vi "Database_UUT - Add UUT.vi"() -> ()   [LabVIEW 2017]
uses:
  Database_UUT_class/TypeDefs/Datatype.ctl
  Database_UUT_class/Database_UUT.lvclass
panel:
  in  "View Part Number":bool
  in  "Part Number:":string="700-001-25"
  in  "Property Values":string[](array[string])
  in  "Datatype":T1[](array[typedef])=[enum."Double", enum."Int32", enum."Double", enum."Double", enum."Double", enum."Double"]
  in  "Property Labels":string[](array[string])=["Rated Current (A)", "Overload Current (%)", "Lower Trip Limit (s)", "Upper Trip Limit (s)", "Maximum Trip Limit (s)", "Cooling Time (s)"]
  in  "View Database":bool
  in  "Quit Program":bool
  in  "Remove From Database":bool
  in  "Verify Path":bool
  in  "Submit Into Database":bool
  in  "TDMS Database File Name:":string="Database"
  in  "Filepath to Directory of Database:":path=path "C:/Users/Test-Eng/Desktop/ATE Development Programing/Database"
  # "TDMS Database Tool Boss 4000"
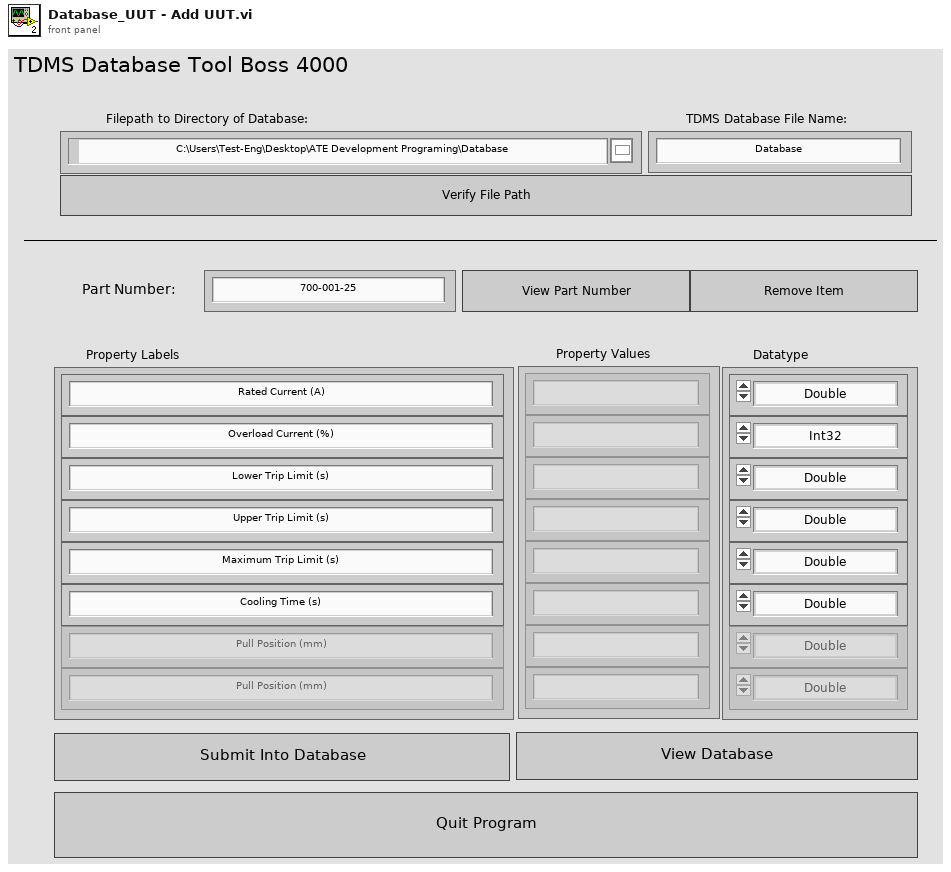
[diagram p1: front panel]
types:
  T1 = typedef "Database_UUT.lvclass/Datatype.ctl" = enum16{"Double", "Int32", "Text String", "Bool (0 or 1)"}
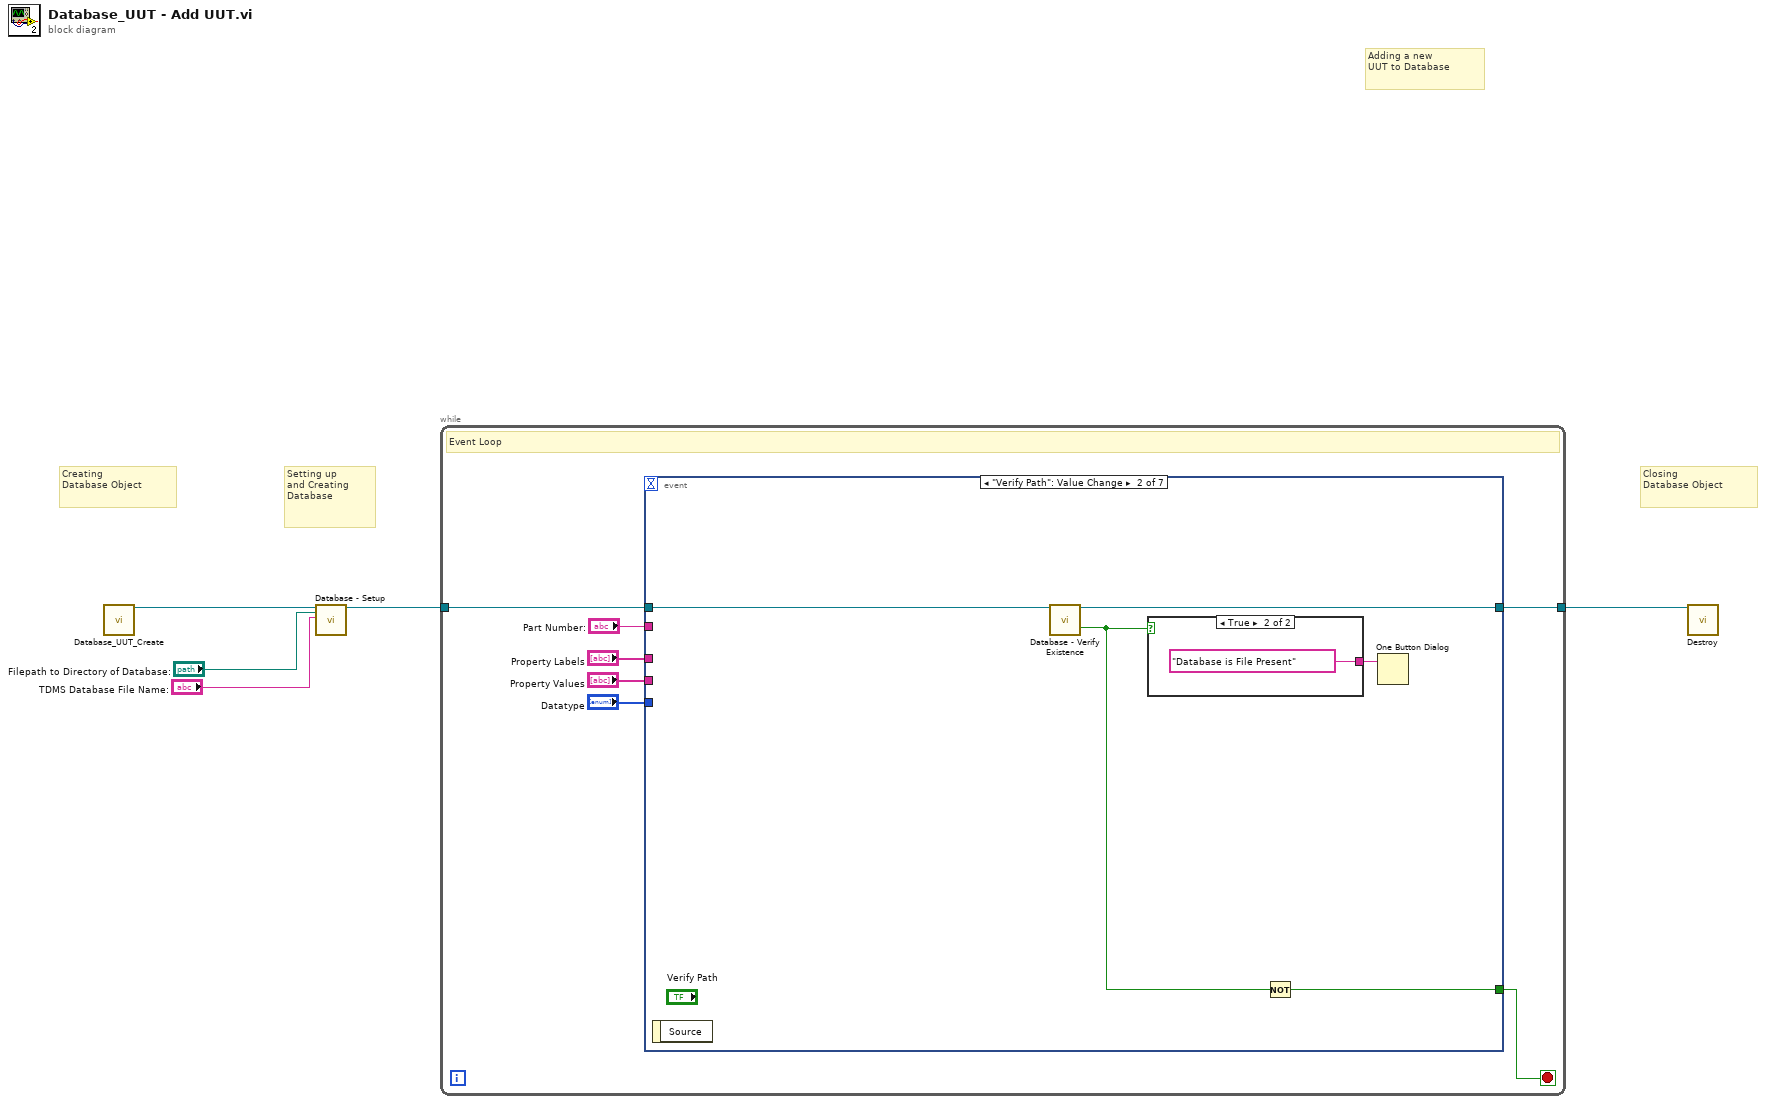
[diagram p0: block diagram]
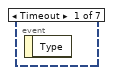
[diagram p2: hidden frame]
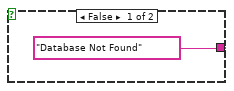
[diagram p3: hidden frame]
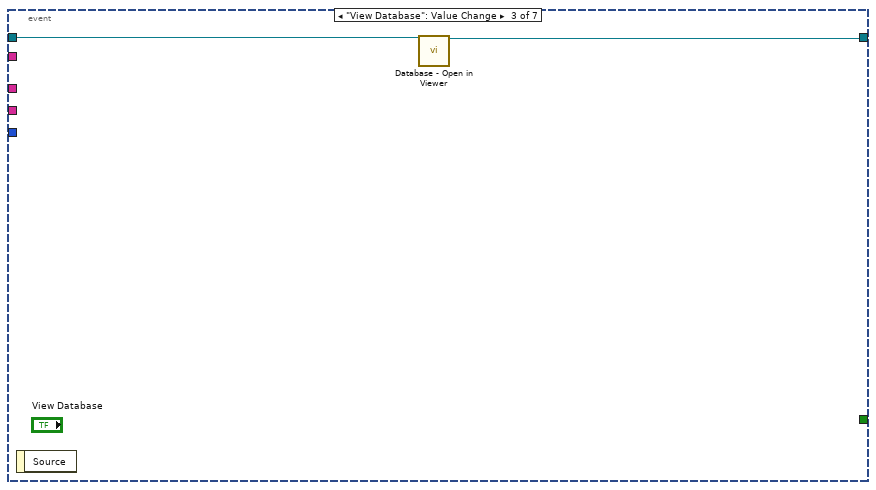
[diagram p4: hidden frame]
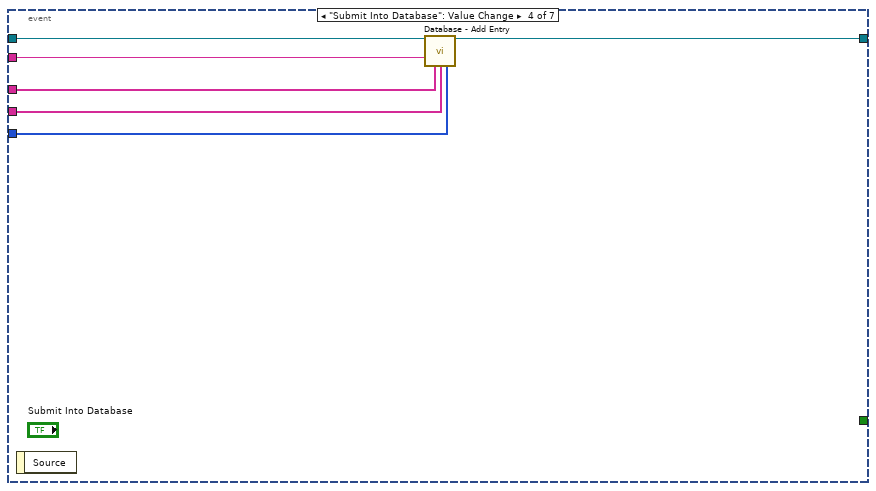
[diagram p5: hidden frame]
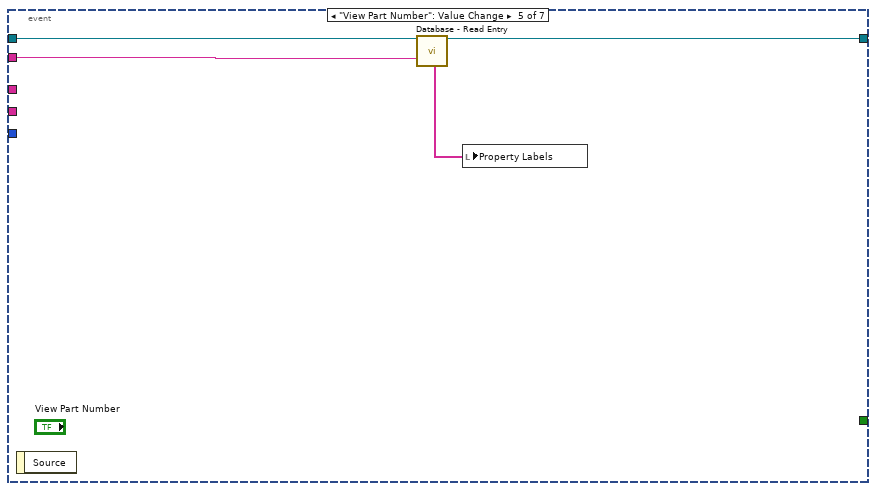
[diagram p6: hidden frame]
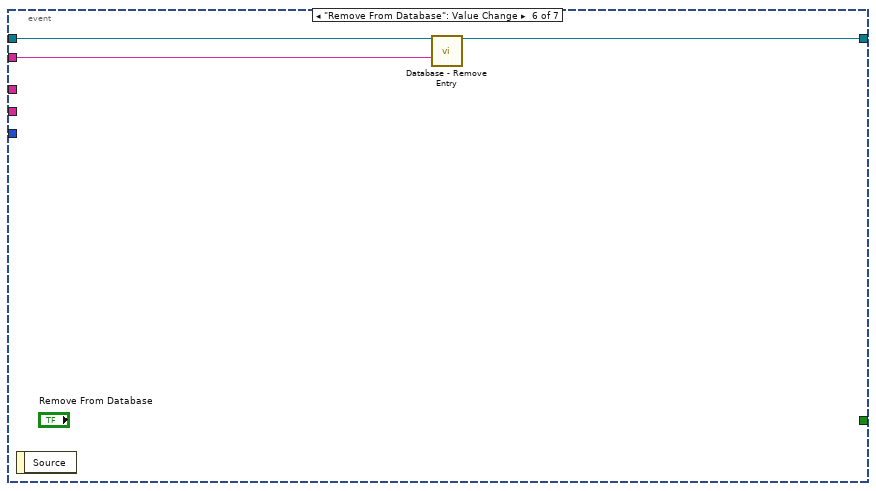
[diagram p7: hidden frame]
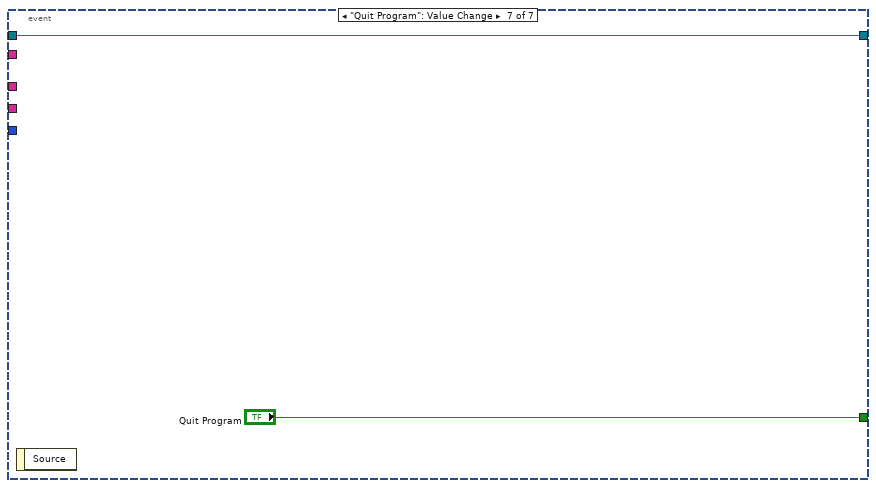
[diagram p8: hidden frame]
diagram:
  # "Closing\nDatabase Object"
  # "Adding a new\nUUT to Database"
  # "Setting up\nand Creating\nDatabase"
  # "Creating\nDatabase Object"
  n1 = call "Database_UUT_Create.vi"() -> ("reference out"=w5:refnum<class "Database_UUT.lvclass">)  [unwired: 18 in, 1 out]
  n2 = call-dynamic "Database - Setup.vi"("reference in"=w5, "Filepath to Directory of Database"="Filepath to Directory of Database:", "Database Name"="TDMS Database File Name:") -> ("reference out"=w2:refnum<class "Database_UUT.lvclass">)  [unwired: 14 in, 2 out]
  n3 = while {
    tunnel: w2 -> [w11]
    tunnel: [w12] -> w1
    stop <- w10 stop-if-true
    # "Event Loop"
    n4 = event shown="[1] \"Verify Path\": Value Change" {
      selector: _ -> [_ _ _ _ _ _ _]
      dyn-events: _ -> [_ _ _ _ _ _ _]
      timeout: _ -> [_ _ _ _ _ _ _]
      tunnel: [_ w16 w20 w26 w30 w34 w35] -> w12
      tunnel: w11 -> [_ w17 w21 w27 w31 w33 w35]
      tunnel: [_ w13 _ _ _ _ "Quit Program"] -> w10
      tunnel: "Part Number:" -> [_ _ _ w25 w29 w32 _]
      tunnel: "Datatype" -> [_ _ _ w24 _ _ _]
      tunnel: "Property Values" -> [_ _ _ w23 _ _ _]
      tunnel: "Property Labels" -> [_ _ _ w22 _ _ _]
      event Timeout {
        n5 = event-data() -> ()  [unwired: 1 in, 1 out]
      }
      event "Verify Path": Value Change {
        n6 = event-data() -> ()  [unwired: 1 in, 1 out]
        n7 = call-dynamic "Database - Verify Existence.vi"("reference in"=w17) -> ("reference out"=w16:refnum<class "Database_UUT.lvclass">, "File Exists/Verified"=w14:bool)  [unwired: 16 in, 1 out]
        n8 = case shown="True" w14 {
          tunnel: ["Database Not Found" "Database is File Present"] -> w15
          frame False {
          }
          frame True {
          }
        }
        n9 = Not(x=w14) -> (.not. x?=w13:bool)
        n10 = One Button Dialog(message=w15) -> ()  [unwired: 1 in, 1 out]
      }
      event "View Database": Value Change {
        n11 = event-data() -> ()  [unwired: 1 in, 1 out]
        n12 = call "Database - Open in Viewer.vi"("reference in"=w21) -> ("reference out"=w20:refnum<class "Database_UUT.lvclass">)  [unwired: 13 in, 1 out]
      }
      event "Submit Into Database": Value Change {
        n13 = event-data() -> ()  [unwired: 1 in, 1 out]
        n14 = call "Database - Add Entry.vi"("reference in"=w27, "Part Number"=w25, "Property Labels"=w22, "Property Values"=w23, "Datatype"=w24) -> ("reference out"=w26:refnum<class "Database_UUT.lvclass">)  [unwired: 9 in, 1 out]
      }
      event "View Part Number": Value Change {
        n15 = event-data() -> ()  [unwired: 1 in, 1 out]
        n16 = call "Database - Read Entry.vi"("reference in"=w31, "Part Number"=w29) -> ("Property Names"=w28:string[], "reference out"=w30:refnum<class "Database_UUT.lvclass">)  [unwired: 11 in, 5 out]
        n17 = local write "Property Labels"(w28) -> ()
      }
      event "Remove From Database": Value Change {
        n18 = event-data() -> ()  [unwired: 1 in, 1 out]
        n19 = call "Database - Remove Entry.vi"("reference in"=w33, "Part Number"=w32) -> ("reference out"=w34:refnum<class "Database_UUT.lvclass">)  [unwired: 12 in, 1 out]
      }
      event "Quit Program": Value Change {
        n20 = event-data() -> ()  [unwired: 1 in, 1 out]
      }
    }
  }
  n21 = call-dynamic "Destroy.vi"("reference in"=w1) -> ()  [unwired: 17 in, 2 out]
